vi "Position Numeric to right of previous.vi"(8 "error in (no error)":errorcluster, 10 "Prev Numeric Ref":refnum<vi>, 11 "Numeric Ref":refnum<vi>) -> (0 "Error Out":errorcluster)   [LabVIEW 2014]
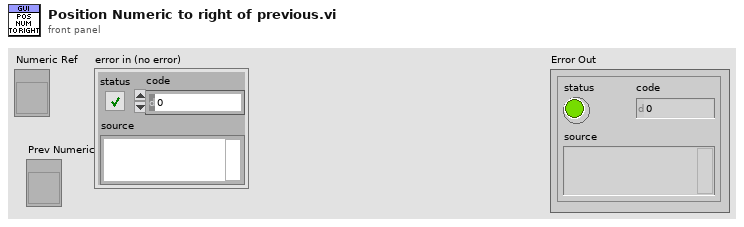
[diagram p1: front panel]
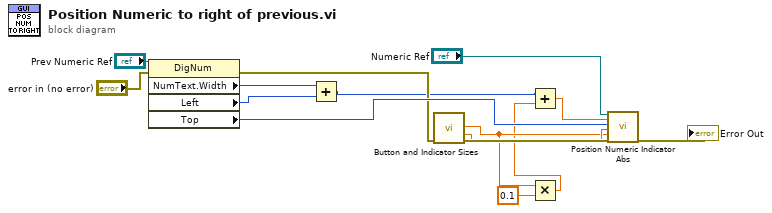
[diagram p0: block diagram]
diagram:
  n1 = property class="DigNum"(reference="Prev Numeric Ref", error in="error in (no error)") -> (error out=w9:errorcluster, "NumText.Width"=w6:u32, "Left"=w11:i32, "Top"=w10:i32)  [unwired: 1 out]
  n2 = Add(x=w6, y=w11) -> (x+y=w3:u32)
  n3 = call "Button and Indicator Sizes.vi"("error in (no error)"=w9) -> ("Numerice Indicator Width"=w5:dbl, "Numeric Indicator Height"=w7:dbl, "error out"=w14:errorcluster)  [unwired: 10 in, 2 out]
  n4 = Multiply(x=w5, y=0.1) -> (x*y=w2:dbl)
  n5 = Add(x=w3, y=w2) -> (x+y=w1:dbl)
  n6 = call "Position Numeric Indicator Abs.vi"("Numeric Ref"="Numeric Ref", "Left Offset (px)"=w1, "Top Offste (px)"=w10, "Height (px)"=w7, "Width (px)"=w5, "Error In"=w14) -> ("Error Out"=→"Error Out":errorcluster)  [unwired: 13 in]
